vi "SIM_CurrentOutput.vi"(9 "array":dbl[][](array[numeric]), 10 "y":dbl, 11 "x":dbl) -> (2 "Zread":dbl)   [LabVIEW 2017]
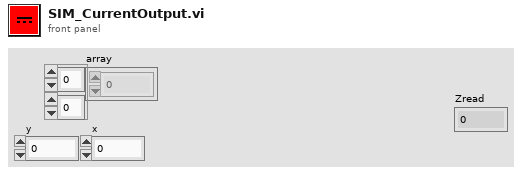
[diagram p1: front panel]
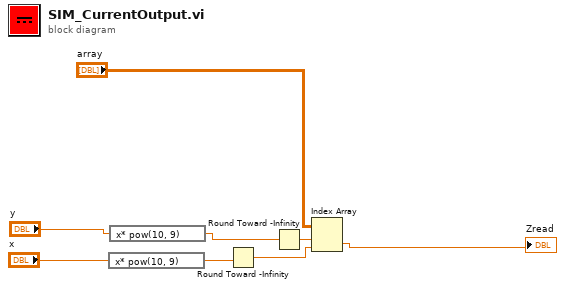
[diagram p0: block diagram]
diagram:
  n1 = expression code="x* pow(10, 9)"("x") -> (w1:dbl)
  n2 = expression code="x* pow(10, 9)"("y") -> (w3:dbl)
  n3 = Round Toward -Infinity(1:w1) -> (0:w7:dbl)
  n4 = Round Toward -Infinity(1:w3) -> (0:w8:dbl)
  n5 = Index Array(array="array", index (row)=w8, index (col)=w7) -> (element=→"Zread":dbl)
